vi "UDPClose.vi"(11 "Double CAN in":T2) -> (0 "Error CAN1":errorcluster {"code" format="%.0x"}, 3 "Error CAN0":errorcluster {"code" format="%.0x"})   [LabVIEW 2017]
uses:
  <vilib>/nican/nican.llb/xobjhandle.ctl
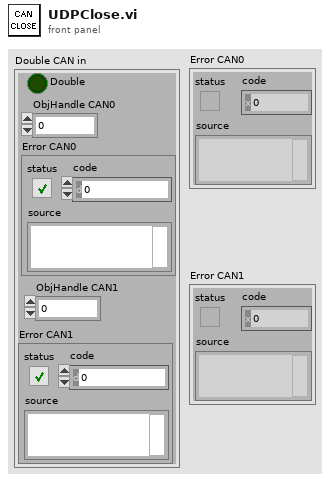
[diagram p1: front panel]
types:
  T1 = typedef "xobjhandle.ctl" = u32
  T2 = cluster{"ObjHandle CAN0":T1, "Error CAN0":errorcluster, "Error CAN1":errorcluster, "ObjHandle CAN1":T1, "Double":bool}
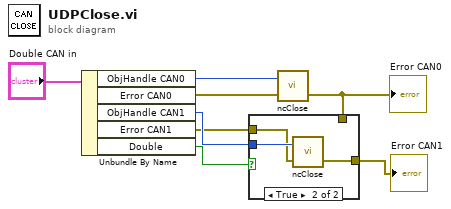
[diagram p0: block diagram]
diagram:
  n1 = Unbundle By Name("Double CAN in") -> ("ObjHandle CAN0"=w7:T1, "Error CAN0"=w6:errorcluster, "ObjHandle CAN1"=w5:T1, "Error CAN1"=w4:errorcluster, "Double"=w1:bool)
  n2 = call <vilib>:"ncClose.vi"("Error in"=w6, "ObjHandle in"=w7) -> ("Error out"=w2:errorcluster)  [unwired: 1 in]
  "Error CAN0" <- w2
  n3 = case shown="True" w1 {
    tunnel: w5 -> [_ w12]
    tunnel: w4 -> [_ w11]
    tunnel: [w9 w10] -> w3
    tunnel: w2 -> [w9 _]
    frame False {
    }
    frame True {
      n4 = call <vilib>:"ncClose.vi"("Error in"=w11, "ObjHandle in"=w12) -> ("Error out"=w10:errorcluster)  [unwired: 1 in]
    }
  }
  "Error CAN1" <- w3
